vi "Rotate Angle in Degrees (Scalar).vi"(7 "output range (-180 to 180)":T1=enum."-180 to 180", 9 "ccw rotation (deg)":dbl, 11 "angle in (deg)":dbl) -> (3 "angle out (deg)":dbl)   [LabVIEW 2017, in "NI_Robotics Utilities.lvlib"]
doc: "This VI is deprecated. Use <vi.lib>\\Analysis\\coordinate.llb\\Angle Rotation.vi instead."
uses:
  <vilib>/robotics/Utilities/NI_Robotics Utilities.lvlib
  <vilib>/robotics/Utilities/Angle Range_Degrees.ctl
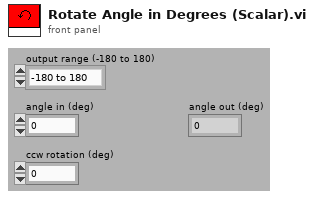
[diagram p1: front panel]
types:
  T1 = typedef "NI_Robotics Utilities.lvlib/Angle Range_Degrees.ctl" = enum16{"none", "-180 to 180", "0 to 360"}
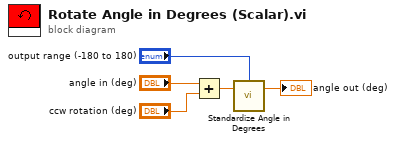
[diagram p0: block diagram]
diagram:
  n1 = Add(x="angle in (deg)", y="ccw rotation (deg)") -> (x+y=w3:dbl)
  n2 = call <vilib>:"Standardize Angle in Degrees.vi"("angle in (deg)"=w3, "range (-180 to 180)"="output range (-180 to 180)") -> ("angle out (deg)"=→"angle out (deg)":dbl)  [unwired: 3 in]
